vi "Actor Core.vi"(8 "error in":errorcluster, 11 "Message Dialog View in":refnum<class "Message Dialog View.lvclass">) -> (0 "error out":errorcluster, 3 "Actor out":refnum<class "Actor.lvclass">)   [LabVIEW 2015, in "Message Dialog View.lvlib" / "Message Dialog View.lvclass"]
doc: "(<B>Filename</B>: Actor Framework.lvlib:Actor.lvclass:Actor Core.vi)\n\nReceives messages to the actor, reacts to them, and initiates any error handling that may shut the actor down.\n\nDescendant classes may override this VI to append parallel tasks for the actor to complete while it handles messages. Overrides use the Call Parent Method node."
uses:
  Message Dialog View.lvclass
  <vilib>/ActorFramework/Actor/Actor.lvclass
  Message Dialog View.lvclass/Message Dialog View.ctl
  <vilib>/ActorFramework/Actor/Actor.lvclass/Actor.ctl
  <vilib>/ActorFramework/Message Enqueuer/Message Enqueuer.lvclass/Message Enqueuer.ctl
  Message Dialog View Messages/Broadcast OK Msg/Broadcast OK Msg.lvclass/Broadcast OK Msg.ctl
  Message Dialog View Messages/Broadcast Cancel Msg/Broadcast Cancel Msg.lvclass/Broadcast Cancel Msg.ctl
  <vilib>/ActorFramework/Message Enqueuer/Init from Existing Queue.vi
  <vilib>/ActorFramework/Message Enqueuer/Enqueue.vi
  <vilib>/ActorFramework/Message Priority Queue/Priority Enqueue.vi
  <vilib>/ActorFrameworkMVC/Abstract View/Abstract View/Abstract View.lvclass
  <vilib>/ActorFramework/Message Enqueuer/Message Enqueuer.lvclass
  Message Dialog View Messages/Broadcast OK Msg/Broadcast OK Msg.lvclass
  Message Dialog View Messages/Broadcast Cancel Msg/Broadcast Cancel Msg.lvclass
panel:
  out "Message":string="Are you sure you want to exit?"
  in  "Cancel Push Button":bool
  in  "OK Push Button":bool
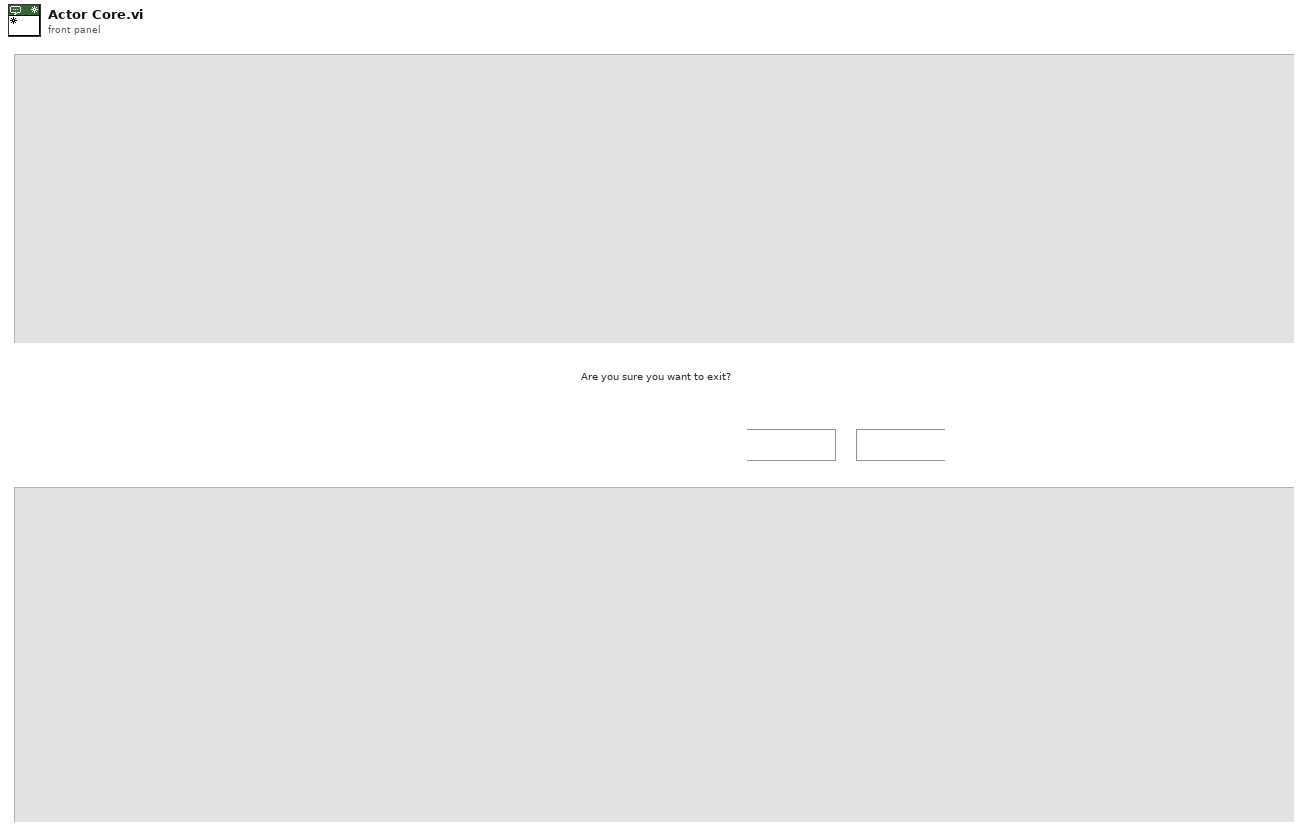
[diagram p1: front panel]
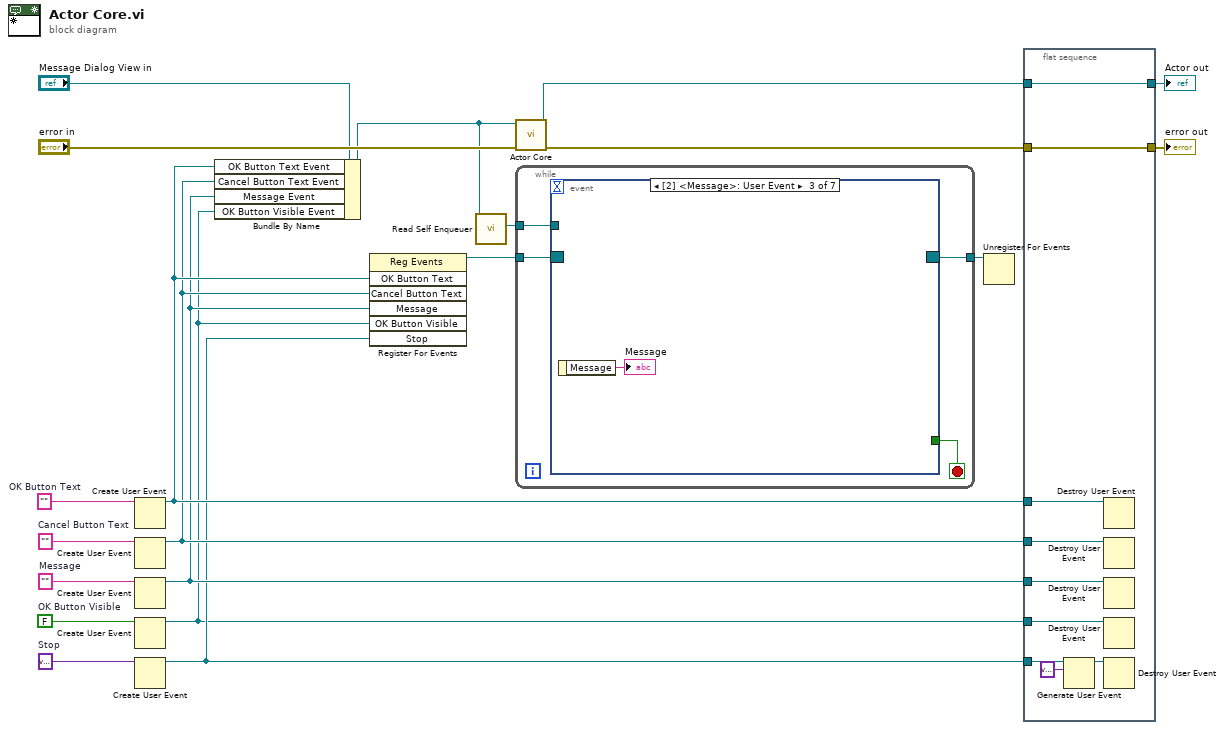
[diagram p0: block diagram]
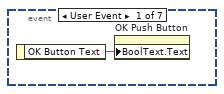
[diagram p2: hidden frame]
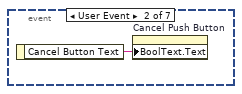
[diagram p3: hidden frame]
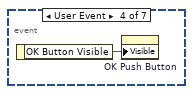
[diagram p4: hidden frame]
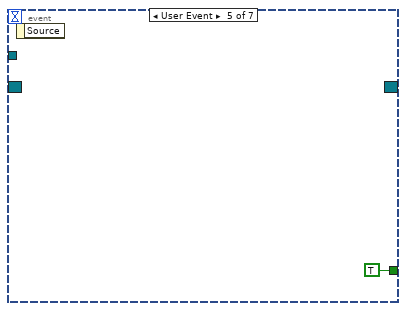
[diagram p5: hidden frame]
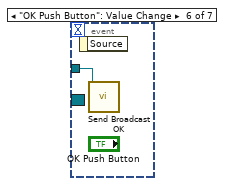
[diagram p6: hidden frame]
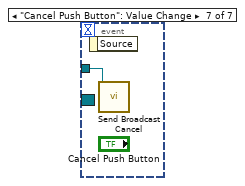
[diagram p7: hidden frame]
diagram:
  w3 = FALSE  # OK Button Visible
  w8 = ""  # Cancel Button Text
  w7 = ""  # OK Button Text
  w14 = variant  # Stop
  w17 = ""  # Message
  n1 = Create User Event(user event datatype=w7) -> (user event=w6:refnum<user-event>)  [unwired: 1 in, 1 out]
  n2 = Create User Event(user event datatype=w8) -> (user event=w5:refnum<user-event>)  [unwired: 1 in, 1 out]
  n3 = Create User Event(user event datatype=w17) -> (user event=w4:refnum<user-event>)  [unwired: 1 in, 1 out]
  n4 = Create User Event(user event datatype=w3) -> (user event=w1:refnum<user-event>)  [unwired: 1 in, 1 out]
  n5 = Create User Event(user event datatype=w14) -> (user event=w2:refnum<user-event>)  [unwired: 1 in, 1 out]
  n6 = Bundle By Name(cluster="Message Dialog View in", "OK Button Text Event"=w6, "Cancel Button Text Event"=w5, "Message Event"=w4, "OK Button Visible Event"=w1) -> (w18:refnum<class "Message Dialog View.lvclass">)
  n7 = register-events(w6, w5, w4, w1, w2) -> (reference out=w15:refnum<event-registration>)  [unwired: 2 in, 1 out]
  n8 = call <vilib>:"Read Self Enqueuer.vi"("Actor"=w18) -> ("Self Enqueuer"=w16:refnum<class "Message Enqueuer.lvclass">)  [unwired: 10 in]
  n9 = call-parent "Actor Core.vi"("error in"="error in", "Abstract View in"=w18) -> ("error out"=w10:errorcluster, "Actor out"=w12:refnum<class "Actor.lvclass">)  [unwired: 8 in]
  n10 = while {
    tunnel: w16 -> [w21]
    tunnel: w15 -> [w24]
    tunnel: [w23] -> w13
    stop <- w22 stop-if-true
    n11 = event shown="[2] <Message>: User Event" {
      selector: w24 -> [_ _ _ _ _ _ _]
      dyn-events: [_ _ _ _ _ _ _] -> w23
      timeout: _ -> [_ _ _ _ _ _ _]
      tunnel: [_ _ _ _ TRUE _ _] -> w22
      tunnel: w21 -> [_ _ _ _ _ w30 w31]
      event User Event {
        n12 = event-data() -> ("OK Button Text"=w25:string)  [unwired: 1 in]
        n13 = property on="OK Push Button" class="Bool (strict)"("BoolText.Text"=w25) -> ()  [unwired: 2 in, 2 out]
      }
      event User Event {
        n14 = event-data() -> ("Cancel Button Text"=w26:string)  [unwired: 1 in]
        n15 = property on="Cancel Push Button" class="Bool (strict)"("BoolText.Text"=w26) -> ()  [unwired: 2 in, 2 out]
      }
      event User Event {
        n16 = event-data() -> ("Message"=→"Message":string)  [unwired: 1 in]
      }
      event User Event {
        n17 = event-data() -> ("OK Button Visible"=w28:bool)  [unwired: 1 in]
        n18 = property on="OK Push Button" class="Bool (strict)"("Visible"=w28) -> ()  [unwired: 2 in, 2 out]
      }
      event User Event {
        n19 = event-data() -> ()  [unwired: 1 in, 1 out]
      }
      event "OK Push Button": Value Change {
        n20 = event-data() -> ()  [unwired: 1 in, 1 out]
        n21 = call "Send Broadcast OK.vi"("Message Enqueuer"=w30) -> ()  [unwired: 9 in, 2 out]
      }
      event "Cancel Push Button": Value Change {
        n22 = event-data() -> ()  [unwired: 1 in, 1 out]
        n23 = call "Send Broadcast Cancel.vi"("Message Enqueuer"=w31) -> ()  [unwired: 9 in, 2 out]
      }
    }
  }
  n24 = Unregister For Events(event registration refnum=w13) -> ()  [unwired: 1 in, 1 out]
  n25 = flat-sequence {
    tunnel: w2 -> [w40]
    tunnel: w4 -> [w37]
    tunnel: w12 -> [w36]
    tunnel: [w36] -> w11
    tunnel: w10 -> [w35]
    tunnel: [w35] -> w9
    tunnel: w6 -> [w34]
    tunnel: w5 -> [w33]
    tunnel: w1 -> [w32]
    frame #0 {
      n26 = Generate User Event(user event=w40, event data cluster=variant ("event data")) -> (user event out=w38:refnum<user-event>)  [unwired: 2 in, 1 out]
      n27 = Destroy User Event(user event=w34) -> ()  [unwired: 1 in, 1 out]
      n28 = Destroy User Event(user event=w33) -> ()  [unwired: 1 in, 1 out]
      n29 = Destroy User Event(user event=w37) -> ()  [unwired: 1 in, 1 out]
      n30 = Destroy User Event(user event=w32) -> ()  [unwired: 1 in, 1 out]
      n31 = Destroy User Event(user event=w38) -> ()  [unwired: 1 in, 1 out]
    }
  }
  "error out" <- w9
  "Actor out" <- w11
